vi "SQLite DB Path.vi"(10 "ping":bool, 11 "database":string="database1.db") -> (3 "Path out":string)   [LabVIEW 2016, in "SQLite Lib.lvlib"]
uses:
  SQLite Lib.lvlib
  <vilib>/Utility/sysdir.llb/System Directory Type.ctl
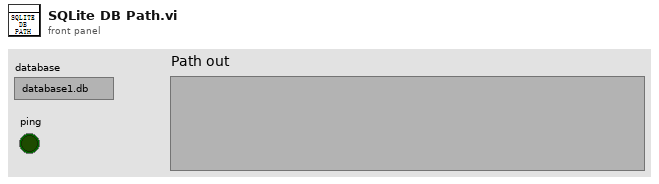
[diagram p1: front panel]
types:
  T1 = typedef "System Directory Type.ctl" = i32
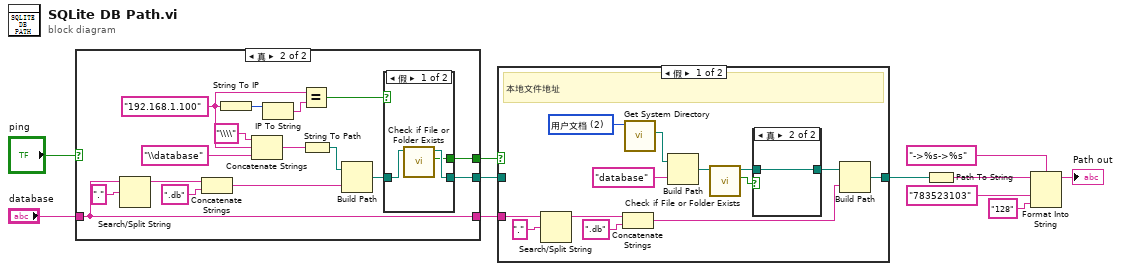
[diagram p0: block diagram]
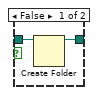
[diagram p2: hidden frame]
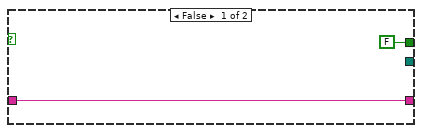
[diagram p4: hidden frame]
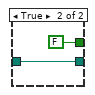
[diagram p5: hidden frame]
diagram:
  n1 = case shown="真" "ping" {
    tunnel: [_ w23] -> w7
    tunnel: [FALSE ("file or folder exists?") w22] -> w9
    tunnel: [w12 w17] -> w8
    tunnel: "database" -> [w12 w17]
    frame False {
    }
    frame True {
      w14 = "192.168.1.100" ("名称")
      n2 = Search/Split String(string=w17, search string/char (-)="." ("搜索字符串/字符(-)")) -> (substring before match=w21:string)  [unwired: 1 in, 2 out]
      n3 = Concatenate Strings(w21, ".db" ("字符串")) -> (w18:string)
      n4 = String To IP(1:w14) -> (0:w29:u32)
      n5 = Concatenate Strings("\\\\" ("字符串"), w14, "\\database" ("名称或相对路径")) -> (w27:string)
      n6 = IP To String(2:w29) -> (0:w26:string)  [unwired: 1 in]
      n7 = Equal?(x=w14, y=w26) -> (x = y?=w25:bool)
      n8 = String To Path(string=w27) -> (path=w15:path)
      n9 = Build Path(base path=w15, name or relative path=w18) -> (appended path=w24:path)
      n10 = case shown="假" w25 {
        tunnel: w24 -> [w32 w33]
        tunnel: [w31 w33] -> w23
        tunnel: [w30 FALSE] -> w22
        frame False {
          n11 = call <vilib>:"Check if File or Folder Exists.vi"("path"=w32) -> ("file or folder exists?"=w30:bool, "dup path"=w31:path)  [unwired: 8 in, 1 out]
        }
        frame True {
        }
      }
    }
  }
  n12 = case shown="假" w9 {
    tunnel: [w47 w51] -> w3
    tunnel: w8 -> [w35 _]
    tunnel: w7 -> [_ w51]
    frame False {
      w39 = T1 2 items=["用户目录"=0, "用户桌面"=1, "用户文档"=2, "用户应用程序数据"=3, "用户设置"=4, "用户临时目录"=5, "公共文档"=6, "公共应用程序数据"=7, "公共设置"=8, "公共缓存"=13, "系统核心库"=9, "系统安装库"=10, "应用程序文件"=11, "启动盘根目录"=12] ("system directory type")
      # "本地文件地址"
      n13 = Search/Split String(string=w35, search string/char (-)="." ("搜索字符串/字符(-)")) -> (substring before match=w43:string)  [unwired: 1 in, 2 out]
      n14 = Concatenate Strings(w43, ".db" ("字符串")) -> (w42:string)
      n15 = call <vilib>:"Get System Directory.vi"("system directory type"=w39) -> ("system directory"=w38:path)  [unwired: 10 in]
      n16 = Build Path(base path=w38, name or relative path="database" ("名称或相对路径")) -> (appended path=w36:path)
      n17 = call <vilib>:"Check if File or Folder Exists.vi"("path"=w36) -> ("file or folder exists?"=w46:bool, "dup path"=w45:path)  [unwired: 8 in, 1 out]
      n18 = case shown="真" w46 {
        tunnel: w45 -> [w49 w50]
        tunnel: [w48 w50] -> w44
        frame False {
          n19 = Create Folder(path (use dialog)=w49) -> (created path=w48:path)  [unwired: 2 in, 2 out]
        }
        frame True {
        }
      }
      n20 = Build Path(base path=w44, name or relative path=w42) -> (appended path=w47:path)
    }
    frame True {
    }
  }
  n21 = Path To String(path=w3) -> (string=w4:string)
  n22 = Format Into String(format string="->%s->%s", initial string=w4, "783523103" ("Enter Password"), "128" ("Enter Password")) -> (resulting string=→"Path out":string)  [unwired: 1 in, 1 out]
